vi "Init.vi"(3 "Container State":T3, 4 "Previous State":variant, 5 "Previous Version":T2) -> (2 "Current State":T1)   [LabVIEW 2021, in "Clock.xctl"]
uses:
  Clock.xctl
  State.ctl
  <resource>/importtools/Common/Event/NISAST Event.lvclass
  <vilib>/_xctls/Container State.ctl
  <vilib>/_xctls/Version.ctl
  update_time.vi
  <vilib>/_xctls/XControlSupport.lvlib
panel:
  in  "Default Indicator State":T1
  in  "Default Control State":T1
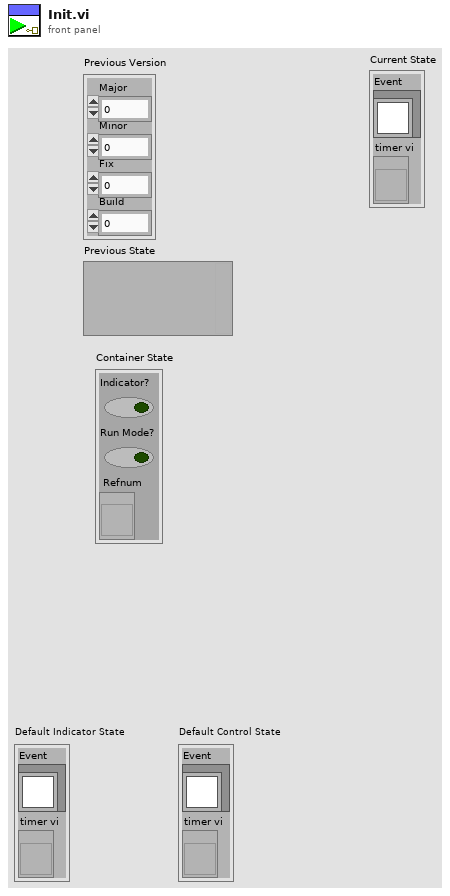
[diagram p1: front panel]
types:
  T1 = typedef "Clock.xctl/State.ctl" = cluster{"Event":refnum<class "NISAST Event.lvclass">, "timer vi":refnum<vi>}
  T2 = typedef "XControlSupport.lvlib/Version.ctl" = cluster{"Major":u16, "Minor":u16, "Fix":u16, "Build":u16}
  T3 = typedef "XControlSupport.lvlib/Container State.ctl" = cluster{"Indicator?":bool, "Run Mode?":bool, " Refnum":refnum<vi>}
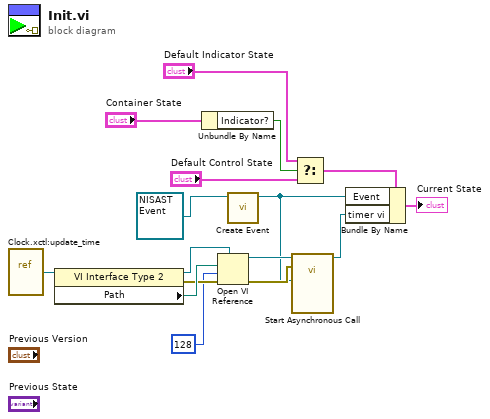
[diagram p0: block diagram]
diagram:
  n1 = vi-ref "Clock.xctl:update_time.vi"() -> (w10:refnum<vi>)
  n2 = property class="VI Interface Type 2"(reference=w10) -> (reference out=w9:refnum<vi>, error out=w6:errorcluster, "Path"=w8:path)  [unwired: 1 in]
  n3 = Unbundle By Name("Container State") -> ("Indicator?"=w13:bool)
  n4 = Open VI Reference(type specifier VI Refnum (for type only)=w9, vi path=w8, options=128, error in (no error)=w6) -> (vi reference=w7:refnum<vi>, error out=w5:errorcluster)  [unwired: 2 in]
  n5 = call-dynamic "Create Event.vi"("Event in"=refnum<class "NISAST Event.lvclass"> refnum) -> ("Event out"=w3:refnum<class "NISAST Event.lvclass">)  [unwired: 8 in, 2 out]
  n6 = call-by-ref "Start Asynchronous Call"(reference=w7, error in=w5, "Event in"=w3) -> (reference out=w2:refnum<vi>)  [unwired: 11 in, 1 out]
  n7 = Select(t="Default Indicator State", s=w13, f="Default Control State") -> (s? t:f=w11:T1)
  n8 = Bundle By Name(cluster=w11, "Event"=w3, "timer vi"=w2) -> (→"Current State":T1)
